vi "Outward.vi"(11 "64 in":refnum<class "Picture.lvclass">) -> (0 "Direction":i32, 1 "Action":T1, 2 "Replicated out":refnum<class "Picture.lvclass">, 3 "64 out":refnum<class "Picture.lvclass">)   [LabVIEW 2020, in "Picture.lvclass"]
uses:
  Picture.lvclass
  Type Defs/Action Enum.ctl
  Type Defs/Direction Enum.ctl
  Picture.lvclass/Picture.ctl
  Type Defs/SB Type Defs.lvlib
  Squares/Common/Common.lvlib
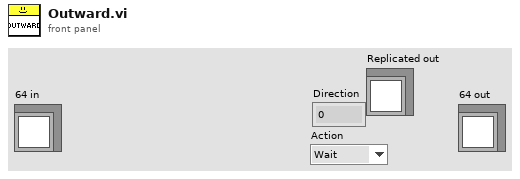
[diagram p1: front panel]
types:
  T1 = typedef "SB Type Defs.lvlib/Action Enum.ctl" = enum16{"Wait", "Move", "Attack", "Replicate"}
  T2 = typedef "SB Type Defs.lvlib/Direction Enum.ctl" = enum16{"NW", "N", "NE", "E", "SE", "S", "SW", "W"}
  T3 = typedef "Common.lvlib/Position.ctl" = cluster{"Column":i32, "Row":i32}
  T4 = typedef "Common.lvlib/Map DVR.ctl" = refnum<data-value>
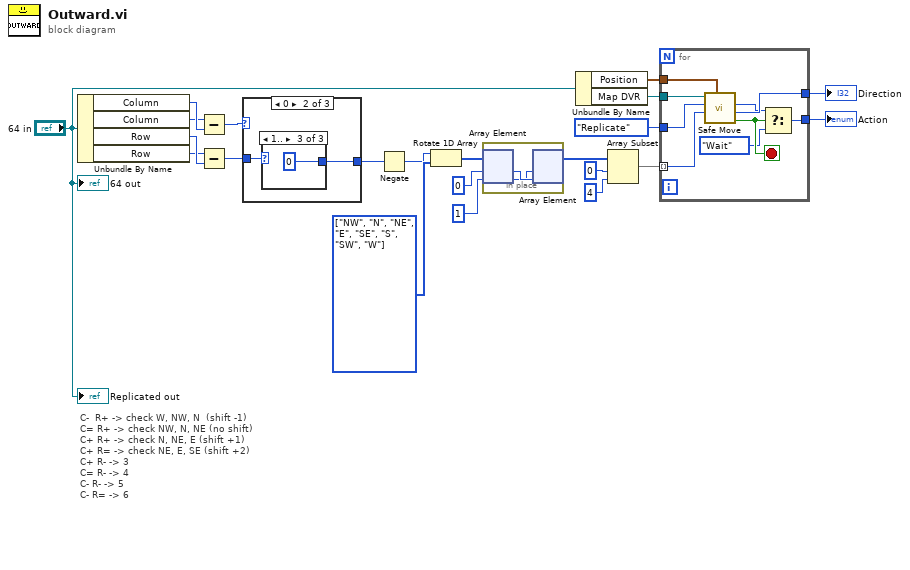
[diagram p0: block diagram]
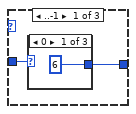
[diagram p2: hidden frame]
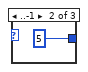
[diagram p3: hidden frame]
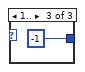
[diagram p4: hidden frame]
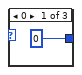
[diagram p5: hidden frame]
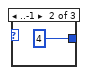
[diagram p6: hidden frame]
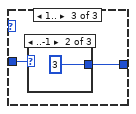
[diagram p7: hidden frame]
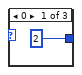
[diagram p8: hidden frame]
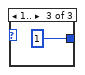
[diagram p9: hidden frame]
diagram:
  w18 = T2[] [enum."NW", enum."N", enum."NE", enum."E", enum."SE", enum."S", enum."SW", enum."W"] items=["NW", "N", "NE", "E", "SE", "S", "SW", "W"]
  # "C-  R+ -> check W, NW, N  (shift -1)\nC= R+ -> check NW, N, NE (no shift)\nC+ R+ -> check N, NE, E (shift +1)\nC+ R= -> check NE, E, SE (shift +2)\nC+ R- -> 3\nC= R- -> 4\nC- R- -> 5\nC- R= -> 6"
  n1 = Unbundle By Name("64 in") -> ("Column"=w22:i32, "Column"=w15:i32, "Row"=w19:i32, "Row"=w16:i32)
  n2 = Subtract(x=w15, y=w22) -> (x-y=w21:i32)
  n3 = Subtract(x=w16, y=w19) -> (x-y=w20:i32)
  n4 = case shown="0" w21 {
    tunnel: w20 -> [w24 w29 w34]
    tunnel: [w23 w28 w33] -> w14
    frame ..-1 {
      n5 = case shown="0" w24 {
        tunnel: [6 5 -1] -> w23
        frame 0 {
        }
        frame ..-1 {
        }
        frame 1.. {
        }
      }
    }
    frame 0 {
      n6 = case shown="1.." w29 {
        tunnel: [0 4 0] -> w28
        frame 0 {
        }
        frame ..-1 {
        }
        frame 1.. {
        }
      }
    }
    frame 1.. {
      n7 = case shown="..-1" w34 {
        tunnel: [2 3 1] -> w33
        frame 0 {
        }
        frame ..-1 {
        }
        frame 1.. {
        }
      }
    }
  }
  n8 = Negate(x=w14) -> (-x=w17:i32)
  n9 = Rotate 1D Array(1:w18, 2:w17) -> (0:w13:T2[])
  n10 = in-place {
    n11 = in-place-array #1(w13, 0, 1) -> (w39:T2, w38:T2)
    n12 = in-place-array #1(w38, w39) -> (w6:T2[])  [unwired: 2 out]
  }
  n13 = Unbundle By Name("64 in") -> ("Position"=w8:T3, "Map DVR"=w10:T4)
  n14 = Array Subset(array=w6, index=0, length=4) -> (w5:T2[])
  n15 = for {
    tunnel: w10 -> [w48]
    tunnel: w8 -> [w47]
    tunnel: Action_Enum."Replicate" ("Desired Action") -> [w46]
    tunnel: w5 -> [w45] mode=indexing
    tunnel: [w44] -> w2
    tunnel: [w40] -> w1
    stop <- w43 stop-if-true
    n16 = call "Safe Move.vi"("Position in"=w47, "Direction in"=w45, "Desired Action"=w46, "Map DVR"=w48) -> ("Accepted?"=w43:bool, "Direction"=w44:T2, "Action"=w41:T1)  [unwired: 4 in, 1 out]
    n17 = Select(t=w41, s=w43, f=Action_Enum."Wait" ("Action")) -> (s? t:f=w40:T1)
  }
  "Direction" <- w2
  "Action" <- w1
  "64 out" <- "64 in"
  "Replicated out" <- "64 in"
